vi "Reward and Action (SubVI).vi"(6 "# each state":i32[](array[numeric])=[1000, 100], 8 "Object":enum16{"Algorithm test", "Flappy Bird"}(ring), 9 "Action":i32, 10 "State":i32, 11 "Q":dbl[][](array[numeric])) -> (2 "Reward":dbl format="%#_13g")   [LabVIEW 2013]
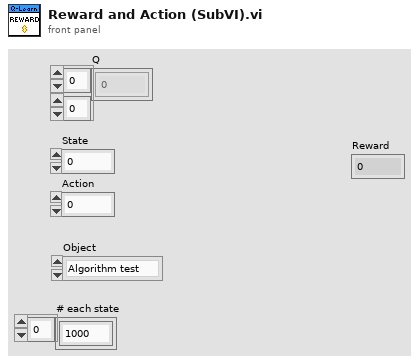
[diagram p1: front panel]
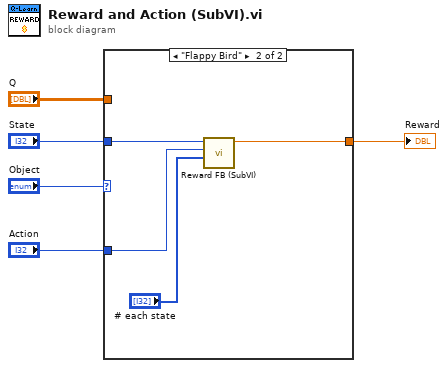
[diagram p0: block diagram]
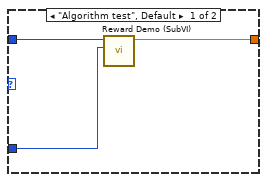
[diagram p2: hidden frame]
diagram:
  n1 = case shown="\"Flappy Bird\"" "Object" {
    tunnel: "State" -> [w8 w12]
    tunnel: "Action" -> [w7 w10]
    tunnel: [w6 w11] -> w2
    tunnel: "Q" -> [_ _]
    frame "Algorithm test", Default {
      n2 = call "Reward Demo (SubVI).vi"("Action"=w7, "State"=w8) -> ("Reward"=w6:dbl)  [unwired: 9 in]
    }
    frame "Flappy Bird" {
      n3 = call "Reward FB (SubVI).vi"("# each state"="# each state", "Action"=w10, "State"=w12) -> ("Reward"=w11:dbl)  [unwired: 8 in]
    }
  }
  "Reward" <- w2
